vi "LED_quickANALYSIS.vi"() -> ()   [LabVIEW 2012]
uses:
  <vilib>/Utility/file.llb/Read From Spreadsheet File (DBL).vi
  <vilib>/gmath/NI_Gmath.lvlib
  <vilib>/Analysis/NI_AALPro.lvlib
panel:
  out "Wavelength":dbl[](array[numeric])
  out "All Counts":dbl[][](array[numeric])
  out "All Abs Irr":dbl[][](array[numeric])
  out "Voltage (Lum)":dbl
  out "Voltage (Cur. Eff.)":dbl
  out "Voltage (EQE)":dbl
  out "Voltage (Lum. Pow. Eff.)":dbl
  in  "Vth_def":dbl=2.1
  out "Von":dbl
  out "Max Cur. Eff.":dbl
  out "Max Lum. Pow. Eff":dbl
  out "Max EQE":dbl
  out "Max Lum.":dbl
  out "Counts/Abs. Irr. vs Wavelength":cluster{"Y":dbl[], "Y":dbl[]}[](graph)
  out "Cur. Eff./Lum. Pow. Eff. vs Voltage":cluster{"Y":dbl[], "Y":dbl[]}[](graph)
  out "Lum. Pow. Eff vs Lum./Cur. Den.":cluster{"Y":dbl[], "Y":dbl[]}[](graph)
  out "Cur. Den. /Lum. vs Voltage":cluster{"Y":dbl[], "Y":dbl[]}[](graph)
  out "Cur. Eff. vs Lum./Cur. Den.":cluster{"Y":dbl[], "Y":dbl[]}[](graph)
  out "x2":dbl=3e-06
  out "x1":dbl=3e-06
  out "WL_1":dbl
  out "WL_2":dbl
  in  "WL_high":dbl=1131.0
  in  "WL_low":dbl=348.0
  out "EQE_array":dbl[](array[numeric])
  out "EQE vs Lum./Cur. Den.":T1(graph)
  out "XY Graph 3":cluster{"Wavelength":dbl[], "Counts":dbl[]}(graph)
  out "Luminance Ratio":dbl[](array[numeric])
  out "Calculated_luminance_array":dbl[](array[numeric])
  out "Calculated_candela_array":dbl[](array[numeric])
  out "Photon_count_array":dbl[](array[numeric])
  out "Photon_count":dbl
  out "Energy_WL":dbl[](array[numeric])
  out "Calculated_candela":dbl
  out "Abs_irr_itpl":dbl[](array[numeric]) format="%_6g"
  out "WL itpl 2":dbl[](array[numeric]) format="%_6g"
  out "Luminous Power Efficiency":dbl[](array[numeric])
  out "current efficiency (Cd/A)":dbl[](array[numeric])
  out "current density (mA/cm2)":dbl[](array[numeric])
  in  "Device Area (m2)":dbl=3e-06
  out "WL_spectrum":dbl[](array[numeric])
  out "Counts_spectrum":dbl[](array[numeric])
  out "Abs_Irr_spectrum":dbl[](array[numeric])
  out "Spectrum":dbl[][](array[numeric])
  out "All Spectrum":dbl[][](array[numeric])
  in  "Spectrum File":path
  out "uW":dbl[](array[numeric])
  out "Luminance":dbl[](array[numeric])
  out "Candela":dbl[](array[numeric])
  out "Current":dbl[](array[numeric])
  out "Voltage":dbl[](array[numeric])
  out "Data":dbl[][](array[numeric]) format="%#.3e"
  in  "Data File":path
  out "max value":dbl
  out "Peak Position":dbl
  out "max index(es)":i32
  out "Iso. Coef. itpl":dbl[](array[numeric]) format="%_6g"
  out "WL itpl":dbl[](array[numeric]) format="%_6g"
  out "XY Graph 2":cluster{"WL":dbl[], "Iso. Coef.":dbl[]}[](graph)
  out "Iso. Coef.":dbl[](array[numeric])
  out "WL":dbl[](array[numeric])
  # "From"
  # "To"
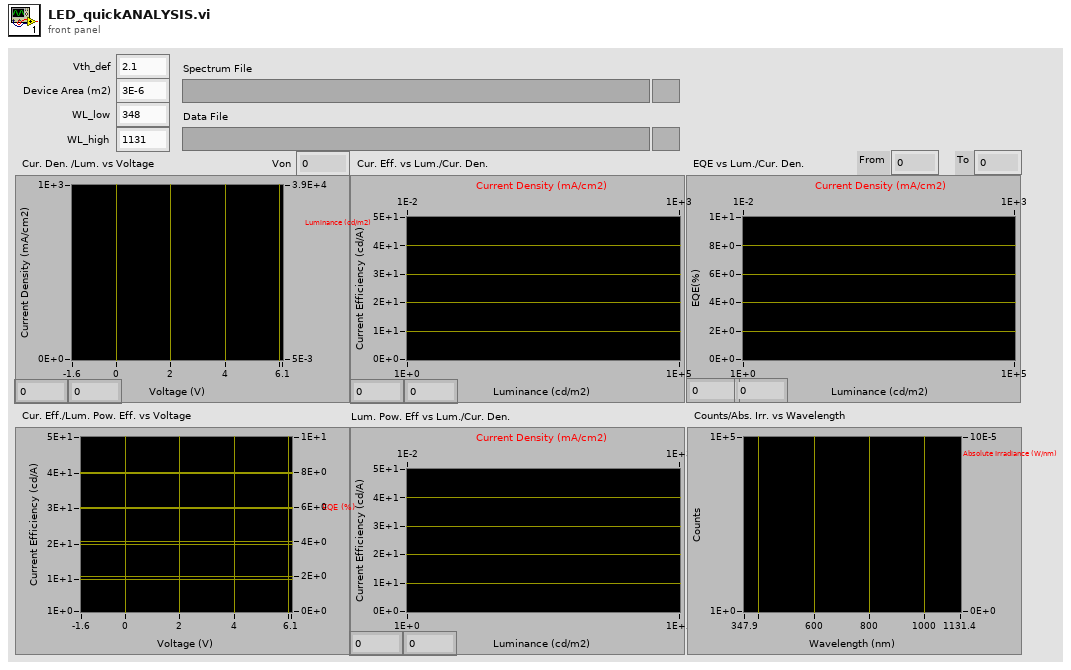
[diagram p1: front panel]
types:
  T1 = cluster{"current density (mA/cm2)":dbl[], "EQE_array":dbl[]}[]
  T2 = cluster{"WL itpl":dbl[], "Iso. Coef. itpl":dbl[]}
  T3 = cluster{"WL itpl":dbl[], "Iso. Coef. itpl":dbl[]}[]
  T4 = cluster{"Luminance":dbl[], "current efficiency (Cd/A)":dbl[]}
  T5 = cluster{"current density (mA/cm2)":dbl[], "current efficiency (Cd/A)":dbl[]}
  T6 = cluster{"current density (mA/cm2)":dbl[], "EQE_array":dbl[]}
  T7 = cluster{"current density (mA/cm2)":dbl[], "current efficiency (Cd/A)":dbl[]}[]
  T8 = cluster{"Voltage":dbl[], "current efficiency (Cd/A)":dbl[]}
  T9 = cluster{"Luminance":dbl[], "Luminous Power Efficiency":dbl[]}
  T10 = cluster{"current density (mA/cm2)":dbl[], "Luminous Power Efficiency":dbl[]}
  T11 = cluster{"current density (mA/cm2)":dbl[], "Luminous Power Efficiency":dbl[]}[]
  T12 = cluster{"WL_spectrum":dbl[], "Counts_spectrum":dbl[]}
  T13 = cluster{"WL_spectrum":dbl[], "Abs_Irr_spectrum":dbl[]}
  T14 = cluster{"WL_spectrum":dbl[], "Abs_Irr_spectrum":dbl[]}[]
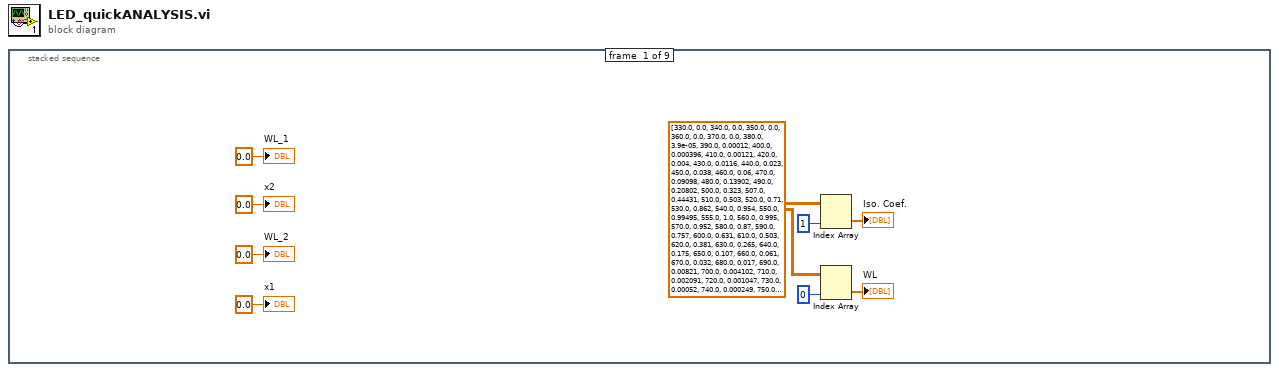
[diagram p0: block diagram]
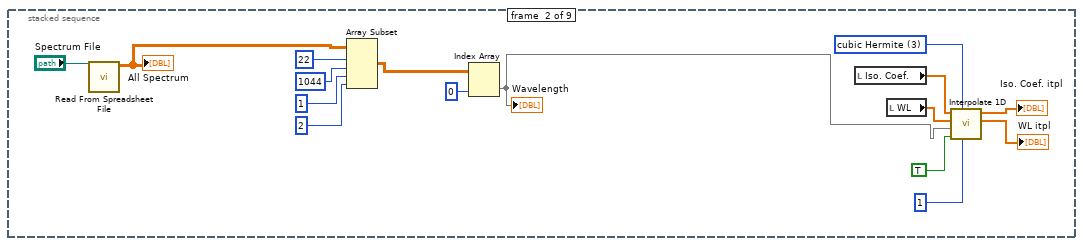
[diagram p2: hidden frame]
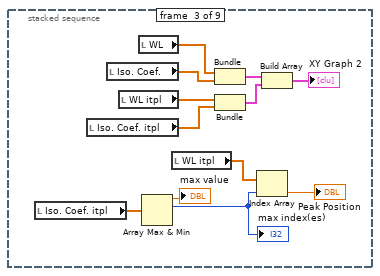
[diagram p3: hidden frame]
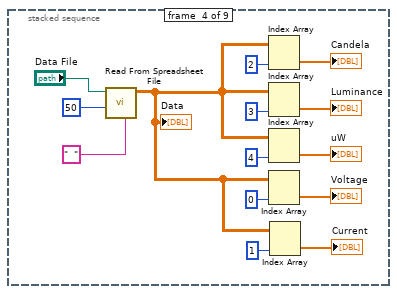
[diagram p4: hidden frame]
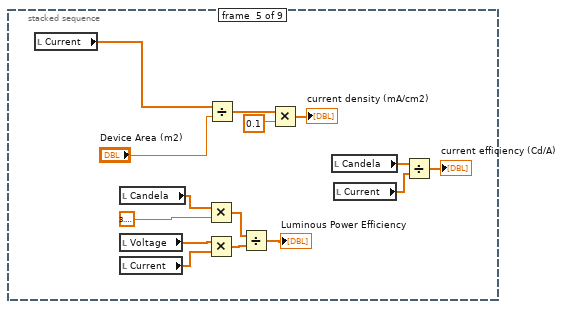
[diagram p5: hidden frame]
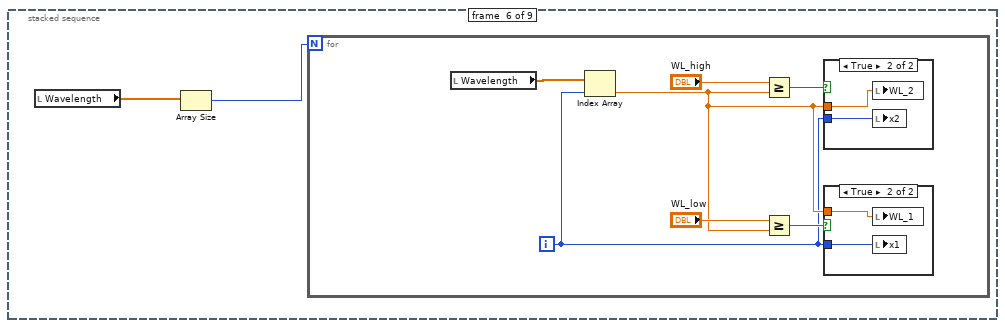
[diagram p6: hidden frame]
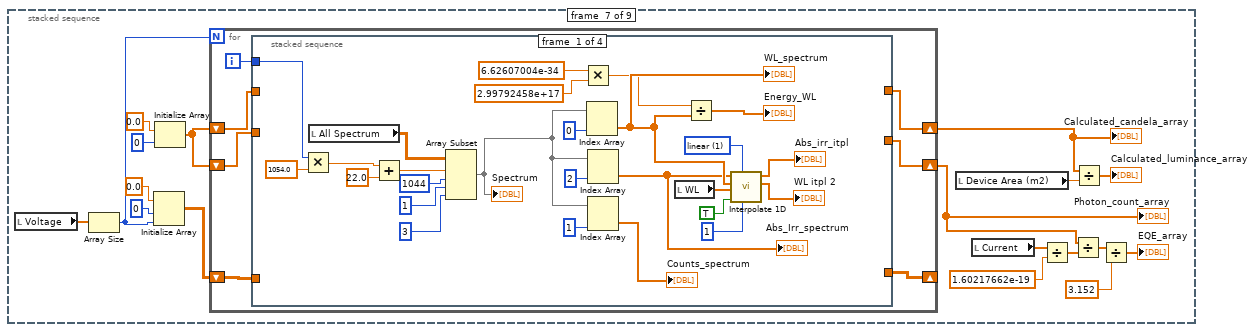
[diagram p9: hidden frame]
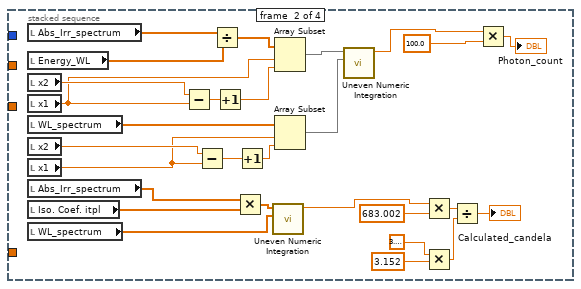
[diagram p10: hidden frame]
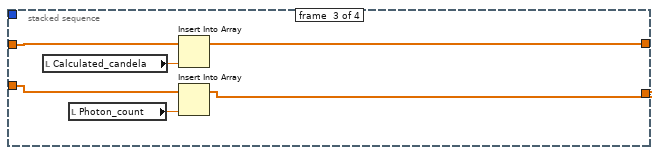
[diagram p11: hidden frame]
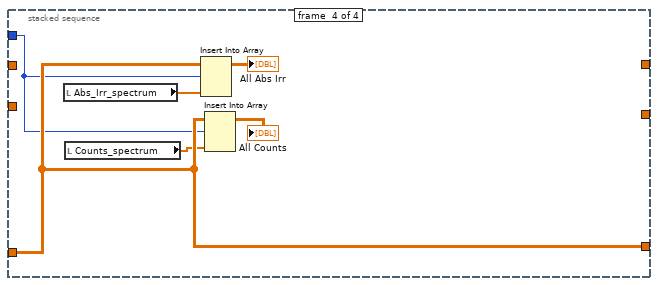
[diagram p12: hidden frame]
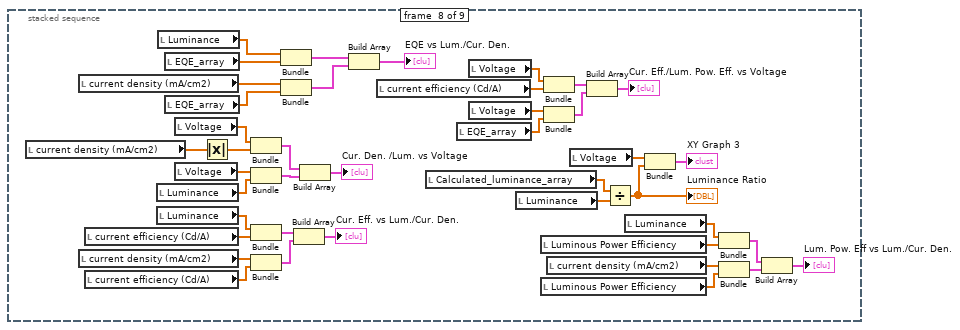
[diagram p13: hidden frame]
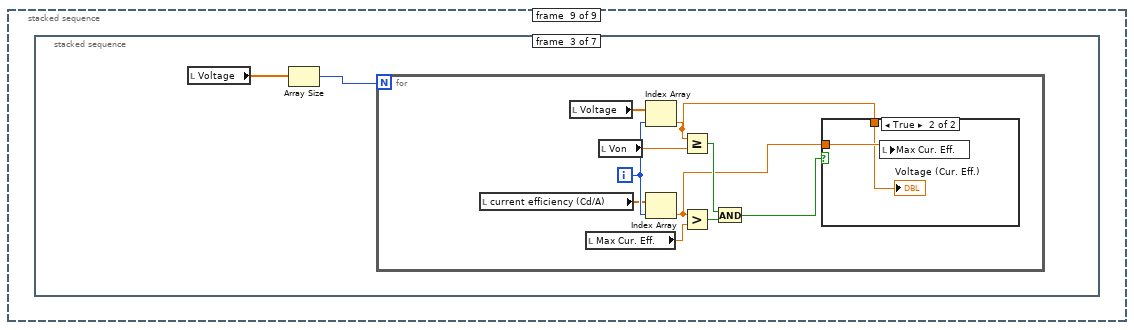
[diagram p14: hidden frame]
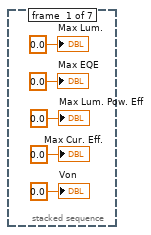
[diagram p15: hidden frame]
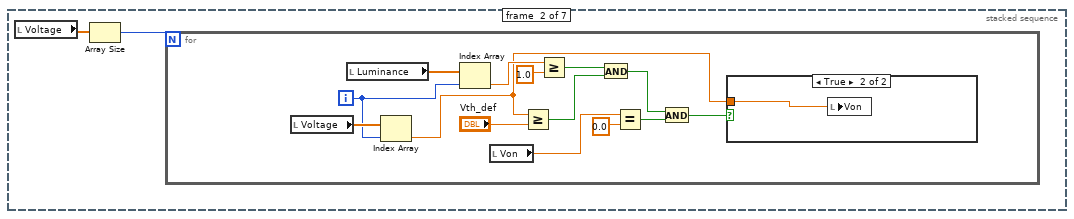
[diagram p16: hidden frame]
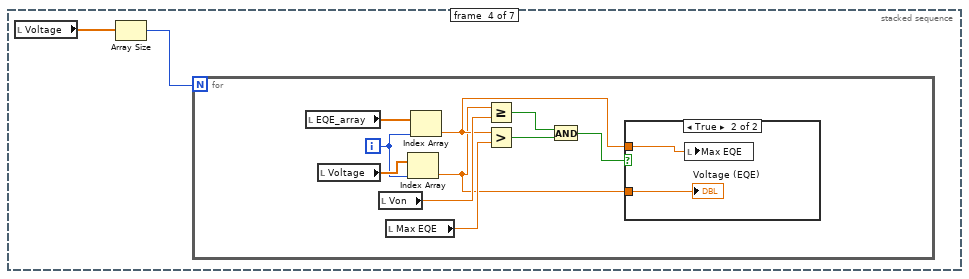
[diagram p19: hidden frame]
diagram:
  n1 = stacked-sequence {
    frame #0 {
      w8 = dbl[][] [[330.0, 0.0], [340.0, 0.0], [350.0, 0.0], [360.0, 0.0], [370.0, 0.0], [380.0, 3.9e-05], [390.0, 0.00012], [400.0, 0.000396], [410.0, 0.00121], [420.0, 0.004], [430.0, 0.0116], [440.0, 0.023], [450.0, 0.038], [460.0, 0.06], [470.0, 0.09098], [480.0, 0.13902], [490.0, 0.20802], [500.0, 0.323], [507.0, 0.44431], [510.0, 0.503], [520.0, 0.71], [530.0, 0.862], [540.0, 0.954], [550.0, 0.99495], [555.0, 1.0], [560.0, 0.995], [570.0, 0.952], [580.0, 0.87], [590.0, 0.757], [600.0, 0.631], [610.0, 0.503], [620.0, 0.381], [630.0, 0.265], [640.0, 0.175], [650.0, 0.107], [660.0, 0.061], [670.0, 0.032], [680.0, 0.017], [690.0, 0.00821], [700.0, 0.004102], [710.0, 0.002091], [720.0, 0.001047], [730.0, 0.00052], [740.0, 0.000249], [750.0, 0.00012], [760.0, 6e-05], [770.0, 3e-05], [780.0, 0.0], [790.0, 0.0], [800.0, 0.0], [810.0, 0.0], [820.0, 0.0], [830.0, 0.0], [840.0, 0.0], [850.0, 0.0], [860.0, 0.0], [870.0, 0.0], [880.0, 0.0], [890.0, 0.0], [900.0, 0.0], [910.0, 0.0], [920.0, 0.0], [930.0, 0.0], [940.0, 0.0], [950.0, 0.0], [960.0, 0.0], [970.0, 0.0], [980.0, 0.0], [990.0, 0.0], [1000.0, 0.0], [1010.0, 0.0], [1020.0, 0.0], [1030.0, 0.0], [1040.0, 0.0], [1050.0, 0.0], [1060.0, 0.0], [1070.0, 0.0], [1080.0, 0.0], [1090.0, 0.0], [1100.0, 0.0], [1110.0, 0.0], [1120.0, 0.0], [1130.0, 0.0], [1140.0, 0.0]] ("all rows")
      n2 = Index Array(array=w8, index (col)=1 ("disabled index (col)")) -> (element=→"Iso. Coef.":dbl[])  [unwired: 1 in]
      n3 = Index Array(array=w8, index (col)=0 ("disabled index (col)")) -> (element=→"WL":dbl[])  [unwired: 1 in]
      "WL_2" <- 0.0 ("WL_2")
      "WL_1" <- 0.0 ("WL_1")
      "x1" <- 0.0 ("x1")
      "x2" <- 0.0 ("x2")
    }
    frame #1 {
      w22 = 3 items=["nearest", "linear", "spline", "cubic Hermite", "Lagrange"] ("method")
      n4 = call-poly <vilib>:"Read From Spreadsheet File.vi"("file path (dialog if empty)"="Spectrum File") -> ("all rows"=w13:dbl[][])  [unwired: 6 in, 4 out]
      "All Spectrum" <- w13
      n5 = Array Subset(array=w13, index (row)=22 ("index"), length (row)=1044 ("length"), index (col)=1 ("index"), length (col)=2 ("length")) -> (w11:dbl[][])
      n6 = Index Array(array=w11, index (col)=0 ("index")) -> (element=w10:dbl[])  [unwired: 1 in]
      "Wavelength" <- w10
      n7 = local read "Iso. Coef."() -> (w24:dbl[])
      n8 = local read "WL"() -> (w25:dbl[])
      n9 = call <vilib>:"Interpolate 1D.vi"("ntimes"=1, "method"=w22, "X is monotonic"=TRUE, "xi"=w10, "X"=w25, "Y"=w24) -> ("xi used"=→"WL itpl":dbl[], "yi"=→"Iso. Coef. itpl":dbl[])  [unwired: 3 in, 1 out]
    }
    frame #2 {
      n10 = local read "Iso. Coef. itpl"() -> (w30:dbl[])
      n11 = local read "Iso. Coef. itpl"() -> (w26:dbl[])
      n12 = local read "Iso. Coef."() -> (w37:dbl[])
      n13 = local read "WL itpl"() -> (w34:dbl[])
      n14 = local read "WL"() -> (w36:dbl[])
      n15 = Array Max & Min(array=w30) -> (max value=→"max value":dbl, max index (indices)=w33:i32)  [unwired: 2 out]
      "max index(es)" <- w33
      n16 = local read "WL itpl"() -> (w32:dbl[])
      n17 = Bundle("WL"=w36, "Iso. Coef."=w37) -> (w35:cluster{"WL":dbl[], "Iso. Coef.":dbl[]})  [unwired: 1 in]
      n18 = Bundle("WL itpl"=w34, "Iso. Coef. itpl"=w26) -> (w27:T2)  [unwired: 1 in]
      n19 = Index Array(array=w32, index=w33) -> (element=→"Peak Position":dbl)
      n20 = Build Array(w35, w27) -> (→"XY Graph 2":T3)
    }
    frame #3 {
      n21 = call-poly <vilib>:"Read From Spreadsheet File.vi"("delimiter (\\t)"="  " ("delimiter (\\t)"), "start of read offset (chars.:0)"=50, "file path (dialog if empty)"="Data File") -> ("all rows"=w39:dbl[][])  [unwired: 4 in, 4 out]
      "Data" <- w39
      n22 = Index Array(array=w39, index (col)=2 ("index (row)")) -> (element=→"Candela":dbl[])  [unwired: 1 in]
      n23 = Index Array(array=w39, index (col)=3 ("index (row)")) -> (element=→"Luminance":dbl[])  [unwired: 1 in]
      n24 = Index Array(array=w39, index (col)=4 ("index (row)")) -> (element=→"uW":dbl[])  [unwired: 1 in]
      n25 = Index Array(array=w39, index (col)=0 ("index (row)")) -> (element=→"Voltage":dbl[])  [unwired: 1 in]
      n26 = Index Array(array=w39, index (col)=1 ("index (row)")) -> (element=→"Current":dbl[])  [unwired: 1 in]
    }
    frame #4 {
      n27 = local read "Current"() -> (w59:dbl[])
      n28 = local read "Candela"() -> (w54:dbl[])
      n29 = local read "Voltage"() -> (w56:dbl[])
      n30 = local read "Current"() -> (w55:dbl[])
      n31 = Multiply(x=w54, y=3.141592653589793) -> (x*y=w57:dbl[])
      n32 = Multiply(x=w56, y=w55) -> (x*y=w58:dbl[])
      n33 = Divide(x=w59, y="Device Area (m2)") -> (x/y=w64:dbl[])
      n34 = Divide(x=w57, y=w58) -> (x/y=→"Luminous Power Efficiency":dbl[])
      n35 = Multiply(x=w64, y=0.1) -> (x*y=→"current density (mA/cm2)":dbl[])
      n36 = local read "Candela"() -> (w61:dbl[])
      n37 = local read "Current"() -> (w62:dbl[])
      n38 = Divide(x=w61, y=w62) -> (x/y=→"current efficiency (Cd/A)":dbl[])
    }
    frame #5 {
      n39 = local read "Wavelength"() -> (w67:dbl[])
      n40 = Array Size(array=w67) -> (size(s)=w68:i32)
      n41 = for {
        N: w68 -> [_]
        i -> [w69]
        n42 = local read "Wavelength"() -> (w71:dbl[])
        n43 = Index Array(array=w71, index=w69) -> (element=w70:dbl)
        n44 = Greater Or Equal?(x="WL_high", y=w70) -> (x >= y?=w73:bool)
        n45 = Greater Or Equal?(x="WL_low", y=w70) -> (x >= y?=w72:bool)
        n46 = case shown="True" w73 {
          tunnel: w70 -> [_ w79]
          tunnel: w69 -> [_ w78]
          frame False {
          }
          frame True {
            n47 = local write "WL_2"(w79) -> ()
            n48 = local write "x2"(w78) -> ()
          }
        }
        n49 = case shown="True" w72 {
          tunnel: w70 -> [_ w77]
          tunnel: w69 -> [_ w76]
          frame False {
          }
          frame True {
            n50 = local write "WL_1"(w77) -> ()
            n51 = local write "x1"(w76) -> ()
          }
        }
      }
    }
    frame #6 {
      n52 = local read "Voltage"() -> (w97:dbl[])
      n53 = Array Size(array=w97) -> (size(s)=w82:i32)
      n54 = Initialize Array(0.0 ("element"), 0 ("dimension size"), w82) -> (w80:dbl[][])
      n55 = Initialize Array(0.0 ("element"), 0 ("dimension size")) -> (w84:dbl[])
      n56 = for {
        N: w82 -> [_]
        shift-right: [w102] -> w94
        shift-left: w84 -> [w103]
        shift-right: [w100] -> w89
        shift-left: w84 -> [w101]
        shift-right: [w98] -> _
        shift-left: w80 -> [w99]
        i -> [w104]
        n57 = stacked-sequence {
          tunnel: w104 -> [w118 _ _ w166]
          tunnel: w103 -> [_ _ w163 _]
          tunnel: [_ _ w162 _] -> w102
          tunnel: w101 -> [_ _ w160 _]
          tunnel: [_ _ w159 _] -> w100
          tunnel: w99 -> [_ _ _ w169]
          tunnel: [_ _ _ w169] -> w98
          frame #0 {
            w115 = 1 items=["nearest", "linear", "spline", "cubic Hermite", "Lagrange"] ("method")
            n58 = Multiply(x=w118, y=1054.0) -> (x*y=w128:dbl)
            n59 = local read "All Spectrum"() -> (w117:dbl[][])
            n60 = Add(x=w128, y=22.0) -> (x+y=w130:dbl)
            n61 = Array Subset(array=w117, index (row)=w130, length (row)=1044 ("length"), index (col)=1 ("index"), length (col)=3 ("length")) -> (w121:dbl[][])
            "Spectrum" <- w121
            n62 = Multiply(x=6.62607004e-34, y=2.99792458e+17) -> (x*y=w108:dbl)
            n63 = Index Array(array=w121, index (col)=0 ("index")) -> (element=w112:dbl[])  [unwired: 1 in]
            "WL_spectrum" <- w112
            n64 = Index Array(array=w121, index (col)=2 ("index")) -> (element=w111:dbl[])  [unwired: 1 in]
            "Abs_Irr_spectrum" <- w111
            n65 = Index Array(array=w121, index (col)=1 ("length")) -> (element=→"Counts_spectrum":dbl[])  [unwired: 1 in]
            n66 = local read "WL"() -> (w110:dbl[])
            n67 = Divide(x=w108, y=w112) -> (x/y=→"Energy_WL":dbl[])
            n68 = call <vilib>:"Interpolate 1D.vi"("ntimes"=1, "method"=w115, "X is monotonic"=TRUE, "xi"=w110, "X"=w112, "Y"=w111) -> ("xi used"=→"WL itpl 2":dbl[], "yi"=→"Abs_irr_itpl":dbl[])  [unwired: 3 in, 1 out]
          }
          frame #1 {
            n69 = local read "Abs_Irr_spectrum"() -> (w150:dbl[])
            n70 = local read "Energy_WL"() -> (w149:dbl[])
            n71 = local read "x2"() -> (w136:dbl)
            n72 = local read "x1"() -> (w135:dbl)
            n73 = local read "WL_spectrum"() -> (w132:dbl[])
            n74 = local read "x2"() -> (w134:dbl)
            n75 = local read "x1"() -> (w133:dbl)
            n76 = local read "Abs_Irr_spectrum"() -> (w158:dbl[])
            n77 = local read "Iso. Coef. itpl"() -> (w157:dbl[])
            n78 = local read "WL_spectrum"() -> (w155:dbl[])
            n79 = Subtract(x=w136, y=w135) -> (x-y=w141:dbl)
            n80 = Subtract(x=w134, y=w133) -> (x-y=w138:dbl)
            n81 = Divide(x=w150, y=w149) -> (x/y=w142:dbl[])
            n82 = Increment(x=w141) -> (x+1=w140:dbl)
            n83 = Multiply(x=w158, y=w157) -> (x*y=w156:dbl[])
            n84 = Increment(x=w138) -> (x+1=w137:dbl)
            n85 = call <vilib>:"Uneven Numeric Integration.vi"("T"=w155, "X"=w156) -> ("result"=w153:dbl)  [unwired: 8 in, 1 out]
            n86 = Array Subset(array=w142, index=w135, length=w140) -> (w139:dbl[])
            n87 = Array Subset(array=w132, index=w133, length=w137) -> (w131:dbl[])
            n88 = call <vilib>:"Uneven Numeric Integration.vi"("T"=w131, "X"=w139) -> ("result"=w148:dbl)  [unwired: 8 in, 1 out]
            n89 = Multiply(x=w153, y=683.002) -> (x*y=w154:dbl)
            n90 = Multiply(x=3.141592653589793, y=3.152) -> (x*y=w144:dbl)
            n91 = Divide(x=w154, y=w144) -> (x/y=→"Calculated_candela":dbl)
            n92 = Multiply(x=w148, y=100.0) -> (x*y=→"Photon_count":dbl)
          }
          frame #2 {
            n93 = local read "Calculated_candela"() -> (w164:dbl)
            n94 = local read "Photon_count"() -> (w161:dbl)
            n95 = Insert Into Array(array=w163, new element=w164) -> (w162:dbl[])  [unwired: 1 in]
            n96 = Insert Into Array(array=w160, new element=w161) -> (w159:dbl[])  [unwired: 1 in]
          }
          frame #3 {
            n97 = local read "Abs_Irr_spectrum"() -> (w170:dbl[])
            n98 = local read "Counts_spectrum"() -> (w168:dbl[])
            n99 = Insert Into Array(array=w169, index (row)=w166, new element=w170) -> (→"All Abs Irr":dbl[][])  [unwired: 1 in]
            n100 = Insert Into Array(array=w169, index (row)=w166, new element=w168) -> (→"All Counts":dbl[][])  [unwired: 1 in]
          }
        }
      }
      "Photon_count_array" <- w89
      "Calculated_candela_array" <- w94
      n101 = local read "Device Area (m2)"() -> (w92:dbl)
      n102 = local read "Current"() -> (w91:dbl[])
      n103 = Divide(x=w91, y=1.60217662e-19) -> (x/y=w90:dbl[])
      n104 = Divide(x=w89, y=w90) -> (x/y=w87:dbl[])
      n105 = Divide(x=w94, y=w92) -> (x/y=→"Calculated_luminance_array":dbl[])
      n106 = Divide(x=w87, y=3.152) -> (x/y=→"EQE_array":dbl[])
    }
    frame #7 {
      n107 = local read "current density (mA/cm2)"() -> (w193:dbl[])
      n108 = local read "current density (mA/cm2)"() -> (w203:dbl[])
      n109 = local read "current density (mA/cm2)"() -> (w186:dbl[])
      n110 = local read "current efficiency (Cd/A)"() -> (w188:dbl[])
      n111 = local read "current efficiency (Cd/A)"() -> (w185:dbl[])
      n112 = local read "Luminance"() -> (w194:dbl[])
      n113 = local read "Luminance"() -> (w187:dbl[])
      n114 = local read "Luminance"() -> (w204:dbl[])
      n115 = local read "EQE_array"() -> (w205:dbl[])
      n116 = local read "EQE_array"() -> (w206:dbl[])
      n117 = local read "Voltage"() -> (w196:dbl[])
      n118 = local read "Voltage"() -> (w195:dbl[])
      n119 = Absolute Value(x=w193) -> (abs(x)=w192:dbl[])
      n120 = Bundle("Voltage"=w196, w192) -> (w199:cluster{"Voltage":dbl[], dbl[]})  [unwired: 1 in]
      n121 = Bundle("Voltage"=w195, "Luminance"=w194) -> (w198:cluster{"Voltage":dbl[], "Luminance":dbl[]})  [unwired: 1 in]
      n122 = Bundle("Luminance"=w187, "current efficiency (Cd/A)"=w188) -> (w191:T4)  [unwired: 1 in]
      n123 = Bundle("current density (mA/cm2)"=w186, "current efficiency (Cd/A)"=w185) -> (w190:T5)  [unwired: 1 in]
      n124 = Bundle("Luminance"=w204, "EQE_array"=w205) -> (w202:cluster{"Luminance":dbl[], "EQE_array":dbl[]})  [unwired: 1 in]
      n125 = Bundle("current density (mA/cm2)"=w203, "EQE_array"=w206) -> (w201:T6)  [unwired: 1 in]
      n126 = Build Array(w191, w190) -> (→"Cur. Eff. vs Lum./Cur. Den.":T7)
      n127 = Build Array(w199, w198) -> (→"Cur. Den. /Lum. vs Voltage":cluster{"Voltage":dbl[], "Luminance":dbl[]}[])
      n128 = Build Array(w202, w201) -> (→"EQE vs Lum./Cur. Den.":T1)
      n129 = local read "current efficiency (Cd/A)"() -> (w172:dbl[])
      n130 = local read "Calculated_luminance_array"() -> (w210:dbl[])
      n131 = local read "EQE_array"() -> (w171:dbl[])
      n132 = local read "Voltage"() -> (w174:dbl[])
      n133 = local read "Voltage"() -> (w173:dbl[])
      n134 = local read "Luminance"() -> (w211:dbl[])
      n135 = local read "Luminous Power Efficiency"() -> (w180:dbl[])
      n136 = local read "Luminous Power Efficiency"() -> (w178:dbl[])
      n137 = Bundle("Voltage"=w174, "current efficiency (Cd/A)"=w172) -> (w177:T8)  [unwired: 1 in]
      n138 = Bundle("Voltage"=w173, "EQE_array"=w171) -> (w176:cluster{"Voltage":dbl[], "EQE_array":dbl[]})  [unwired: 1 in]
      n139 = local read "current density (mA/cm2)"() -> (w179:dbl[])
      n140 = local read "Voltage"() -> (w209:dbl[])
      n141 = Build Array(w177, w176) -> (→"Cur. Eff./Lum. Pow. Eff. vs Voltage":cluster{"Voltage":dbl[], "EQE_array":dbl[]}[])
      n142 = Divide(x=w210, y=w211) -> (x/y=w208:dbl[])
      "Luminance Ratio" <- w208
      n143 = local read "Luminance"() -> (w181:dbl[])
      n144 = Bundle("Voltage"=w209, w208) -> (→"XY Graph 3":cluster{"Voltage":dbl[], dbl[]})  [unwired: 1 in]
      n145 = Bundle("Luminance"=w181, "Luminous Power Efficiency"=w180) -> (w184:T9)  [unwired: 1 in]
      n146 = Bundle("current density (mA/cm2)"=w179, "Luminous Power Efficiency"=w178) -> (w183:T10)  [unwired: 1 in]
      n147 = Build Array(w184, w183) -> (→"Lum. Pow. Eff vs Lum./Cur. Den.":T11)
    }
    frame #8 {
      n148 = stacked-sequence {
        frame #0 {
          "Max Lum." <- 0.0 ("element")
          "Max EQE" <- 0.0 ("element")
          "Max Lum. Pow. Eff" <- 0.0 ("element")
          "Max Cur. Eff." <- 0.0 ("element")
          "Von" <- 0.0 ("element")
        }
        frame #1 {
          n149 = local read "Voltage"() -> (w217:dbl[])
          n150 = Array Size(array=w217) -> (size(s)=w218:i32)
          n151 = for {
            N: w218 -> [_]
            i -> [w228]
            n152 = local read "Voltage"() -> (w230:dbl[])
            n153 = local read "Luminance"() -> (w229:dbl[])
            n154 = Index Array(array=w230, index=w228) -> (element=w219:dbl)
            n155 = Index Array(array=w229, index=w228) -> (element=w227:dbl)
            n156 = local read "Von"() -> (w224:dbl)
            n157 = Greater Or Equal?(x=w219, y="Vth_def") -> (x >= y?=w232:bool)
            n158 = Greater Or Equal?(x=w227, y=1.0) -> (x >= y?=w225:bool)
            n159 = And(x=w225, y=w232) -> (x .and. y?=w221:bool)
            n160 = Equal?(x=w224, y=0.0) -> (x = y?=w222:bool)
            n161 = And(x=w221, y=w222) -> (x .and. y?=w220:bool)
            n162 = case shown="True" w220 {
              tunnel: w219 -> [_ w233]
              frame False {
              }
              frame True {
                n163 = local write "Von"(w233) -> ()
              }
            }
          }
        }
        frame #2 {
          n164 = local read "Voltage"() -> (w234:dbl[])
          n165 = Array Size(array=w234) -> (size(s)=w235:i32)
          n166 = for {
            N: w235 -> [_]
            i -> [w241]
            n167 = local read "current efficiency (Cd/A)"() -> (w240:dbl[])
            n168 = local read "Voltage"() -> (w245:dbl[])
            n169 = local read "Max Cur. Eff."() -> (w242:dbl)
            n170 = local read "Von"() -> (w244:dbl)
            n171 = Index Array(array=w245, index=w241) -> (element=w236:dbl)
            n172 = Index Array(array=w240, index=w241) -> (element=w237:dbl)
            n173 = Greater Or Equal?(x=w236, y=w244) -> (x >= y?=w243:bool)
            n174 = Greater?(x=w237, y=w242) -> (0:w239:bool)
            n175 = And(x=w243, y=w239) -> (x .and. y?=w238:bool)
            n176 = case shown="True" w238 {
              tunnel: w237 -> [_ w247]
              tunnel: w236 -> [_ w246]
              frame False {
              }
              frame True {
                n177 = local write "Max Cur. Eff."(w247) -> ()
                "Voltage (Cur. Eff.)" <- w246
              }
            }
          }
        }
        frame #3 {
          n178 = local read "Voltage"() -> (w248:dbl[])
          n179 = Array Size(array=w248) -> (size(s)=w249:i32)
          n180 = for {
            N: w249 -> [_]
            i -> [w255]
            n181 = local read "EQE_array"() -> (w254:dbl[])
            n182 = local read "Voltage"() -> (w259:dbl[])
            n183 = local read "Von"() -> (w258:dbl)
            n184 = local read "Max EQE"() -> (w256:dbl)
            n185 = Index Array(array=w259, index=w255) -> (element=w250:dbl)
            n186 = Index Array(array=w254, index=w255) -> (element=w251:dbl)
            n187 = Greater Or Equal?(x=w250, y=w258) -> (x >= y?=w257:bool)
            n188 = Greater?(x=w251, y=w256) -> (0:w253:bool)
            n189 = And(x=w257, y=w253) -> (x .and. y?=w252:bool)
            n190 = case shown="True" w252 {
              tunnel: w251 -> [_ w261]
              tunnel: w250 -> [_ w260]
              frame False {
              }
              frame True {
                n191 = local write "Max EQE"(w261) -> ()
                "Voltage (EQE)" <- w260
              }
            }
          }
        }
        frame #4 {
          n192 = local read "Voltage"() -> (w262:dbl[])
          n193 = Array Size(array=w262) -> (size(s)=w263:i32)
          n194 = for {
            N: w263 -> [_]
            i -> [w269]
            n195 = local read "Luminous Power Efficiency"() -> (w268:dbl[])
            n196 = local read "Max Lum. Pow. Eff"() -> (w270:dbl)
            n197 = local read "Voltage"() -> (w273:dbl[])
            n198 = local read "Von"() -> (w272:dbl)
            n199 = Index Array(array=w273, index=w269) -> (element=w264:dbl)
            n200 = Index Array(array=w268, index=w269) -> (element=w265:dbl)
            n201 = Greater Or Equal?(x=w264, y=w272) -> (x >= y?=w271:bool)
            n202 = Greater?(x=w265, y=w270) -> (0:w267:bool)
            n203 = And(x=w271, y=w267) -> (x .and. y?=w266:bool)
            n204 = case shown="True" w266 {
              tunnel: w265 -> [_ w275]
              tunnel: w264 -> [_ w274]
              frame False {
              }
              frame True {
                n205 = local write "Max Lum. Pow. Eff"(w275) -> ()
                "Voltage (Lum. Pow. Eff.)" <- w274
              }
            }
          }
        }
        frame #5 {
          n206 = local read "Voltage"() -> (w276:dbl[])
          n207 = Array Size(array=w276) -> (size(s)=w277:i32)
          n208 = for {
            N: w277 -> [_]
            i -> [w283]
            n209 = local read "Luminance"() -> (w282:dbl[])
            n210 = local read "Voltage"() -> (w287:dbl[])
            n211 = local read "Von"() -> (w286:dbl)
            n212 = local read "Max Lum."() -> (w284:dbl)
            n213 = Index Array(array=w287, index=w283) -> (element=w278:dbl)
            n214 = Index Array(array=w282, index=w283) -> (element=w279:dbl)
            n215 = Greater Or Equal?(x=w278, y=w286) -> (x >= y?=w285:bool)
            n216 = Greater?(x=w279, y=w284) -> (0:w281:bool)
            n217 = And(x=w285, y=w281) -> (x .and. y?=w280:bool)
            n218 = case shown="True" w280 {
              tunnel: w279 -> [_ w289]
              tunnel: w278 -> [_ w288]
              frame False {
              }
              frame True {
                n219 = local write "Max Lum."(w289) -> ()
                "Voltage (Lum)" <- w288
              }
            }
          }
        }
        frame #6 {
          n220 = local read "Counts_spectrum"() -> (w291:dbl[])
          n221 = local read "Abs_Irr_spectrum"() -> (w290:dbl[])
          n222 = local read "WL_spectrum"() -> (w292:dbl[])
          n223 = local read "WL_spectrum"() -> (w293:dbl[])
          n224 = Bundle("WL_spectrum"=w292, "Counts_spectrum"=w291) -> (w296:T12)  [unwired: 1 in]
          n225 = Bundle("WL_spectrum"=w293, "Abs_Irr_spectrum"=w290) -> (w295:T13)  [unwired: 1 in]
          n226 = Build Array(w296, w295) -> (→"Counts/Abs. Irr. vs Wavelength":T14)
        }
      }
    }
  }
